vi "cryotrigger.vi"() -> ()   [LabVIEW 2012]
uses:
  <vilib>/Instr/_visa.llb/VISA Configure Serial Port (Instr).vi
panel:
  in  "VISA resource name":refnum<visa-resource-name>="COM5"
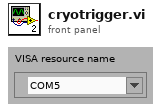
[diagram p1: front panel]
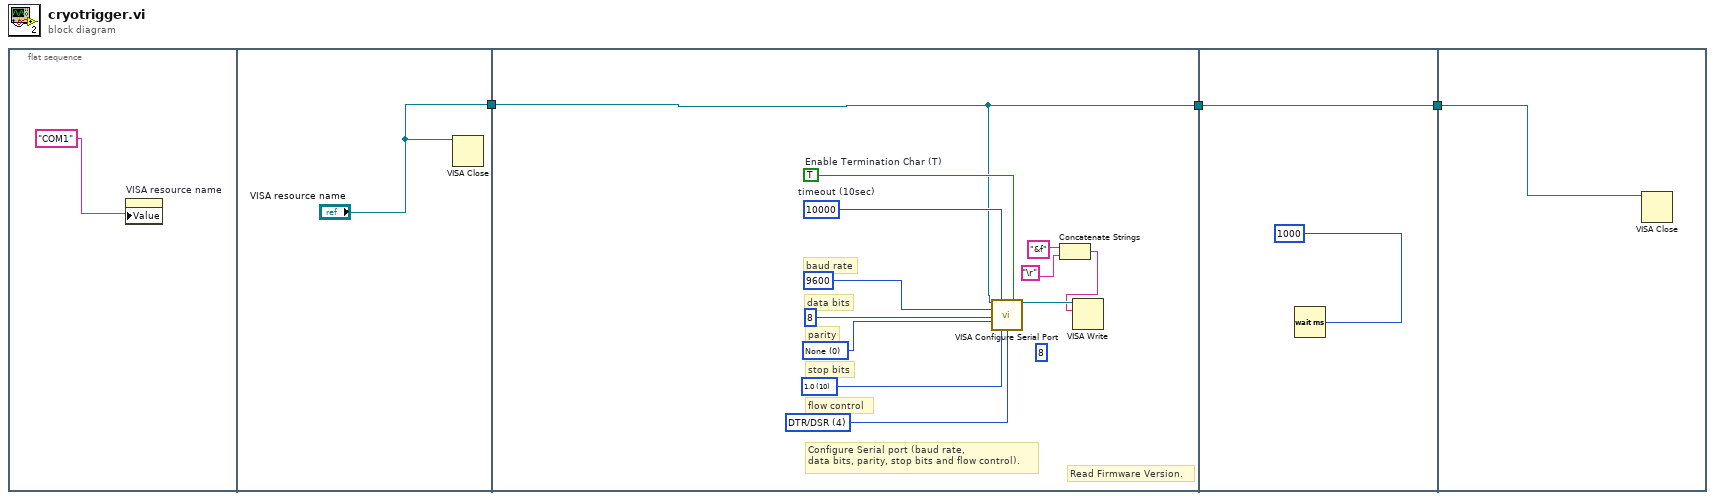
[diagram p0: block diagram]
diagram:
  n1 = flat-sequence {
    tunnel: ["VISA resource name"] -> w3
    tunnel: w3 -> [w6]
    tunnel: [w6] -> w1
    tunnel: [w18] -> w2
    tunnel: w1 -> [w18]
    tunnel: w2 -> [w20]
    frame #0 {
      n2 = property on="VISA resource name" class="VISAName"("Value"="COM1") -> ()  [unwired: 2 in, 2 out]
    }
    frame #1 {
      n3 = VISA Close(VISA resource name="VISA resource name") -> ()  [unwired: 1 in, 1 out]
    }
    frame #2 {
      (unwired) 8
      w11 = u16 4 items=["None"=0, "XON/XOFF"=1, "RTS/CTS"=2, "DTR/DSR"=4] ("flow control")
      w12 = u16 10 items=["1.0"=10, "1.5"=15, "2.0"=20] ("stop bits")
      w13 = u16 0 items=["None", "Odd", "Even", "Mark", "Space"] ("parity")
      w16 = TRUE  # Enable Termination Char (T)
      w17 = u32 10000  # timeout (10sec)
      # "Read Firmware Version."
      # "flow control"
      # "stop bits"
      # "parity"
      # "data bits"
      # "baud rate"
      # "Configure Serial port (baud rate,\ndata bits, parity, stop bits and flow control)."
      n4 = call-poly "VISA Configure Serial Port"("VISA resource name"=w6, "timeout (10sec)"=w17, "Enable Termination\nChar (T)"=w16, "baud rate (9600)"=u32 9600 ("baud rate"), "data bits (8)"=u16 8 ("data bits"), "parity (0:none)"=w13, "stop bits (10: 1 bit)"=w12, "flow control (0:none)"=w11) -> ("VISA resource name out"=w8:refnum<visa-resource-name>)  [unwired: 1 in, 6 out]
      n5 = Concatenate Strings("&f" ("write buffer"), "\r") -> (w7:string)
      n6 = VISA Write(VISA resource name=w8, write buffer=w7) -> ()  [unwired: 1 in, 3 out]
    }
    frame #3 {
      n7 = Wait (ms)(milliseconds to wait=1000) -> ()  [unwired: 1 out]
    }
    frame #4 {
      n8 = VISA Close(VISA resource name=w20) -> ()  [unwired: 1 in, 1 out]
    }
  }
